vi "SMS Analysis Interface.vi"(7 "Calling VI Ref":refnum<vi>) -> ()   [LabVIEW 2016]
uses:
  <vilib>/Utility/miscctls.llb/LVPointTypeDef.ctl
  Orca Flash Data Spooler/Orca Data Spooler Type Defs/Orca Data Spooler Transfer Data.ctl
  SMS Analysis Interface Type Defs/SMS Analysis Interface Connection Info.ctl
panel:
  in  "Clear Queue":bool
  out "Connection Error":bool
  out "Remote Running":bool
  out "Remote Ready":bool
  in  "Queue List":i32(listbox)
  in  "Pause Queue":bool
  in  "Quit Remote":bool
  in  "Add Dataset":bool
  in  "Quit":bool
  out "Start Up Error":errorcluster
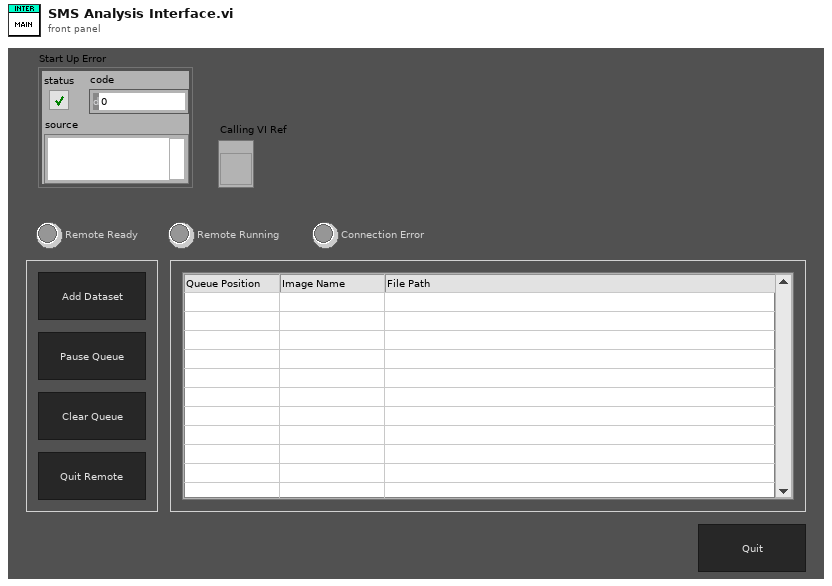
[diagram p1: front panel]
types:
  T1 = typedef "SMS Analysis Interface Connection Info.ctl" = cluster{"Remote IP":string, "Port":u16}
  T2 = typedef "Orca Data Spooler Transfer Data.ctl" = cluster{"transLogPath":string, "imageName":string, "noFrames":u32, "noCycles":u16, "quitFlag":bool}
  T3 = enum16{"Always On", "Always Off", "Off While Running"}
  T4 = typedef "LVPointTypeDef.ctl" = cluster{"Horizontal":i16, "Vertical":i16}
  T5 = typedef "LVRectTypeDef.ctl" = cluster{"Left":i16, "Top":i16, "Right":i16, "Bottom":i16}
  T6 = typedef "LVBoundsTypeDef.ctl" = cluster{"Width":u32, "Height":u32}
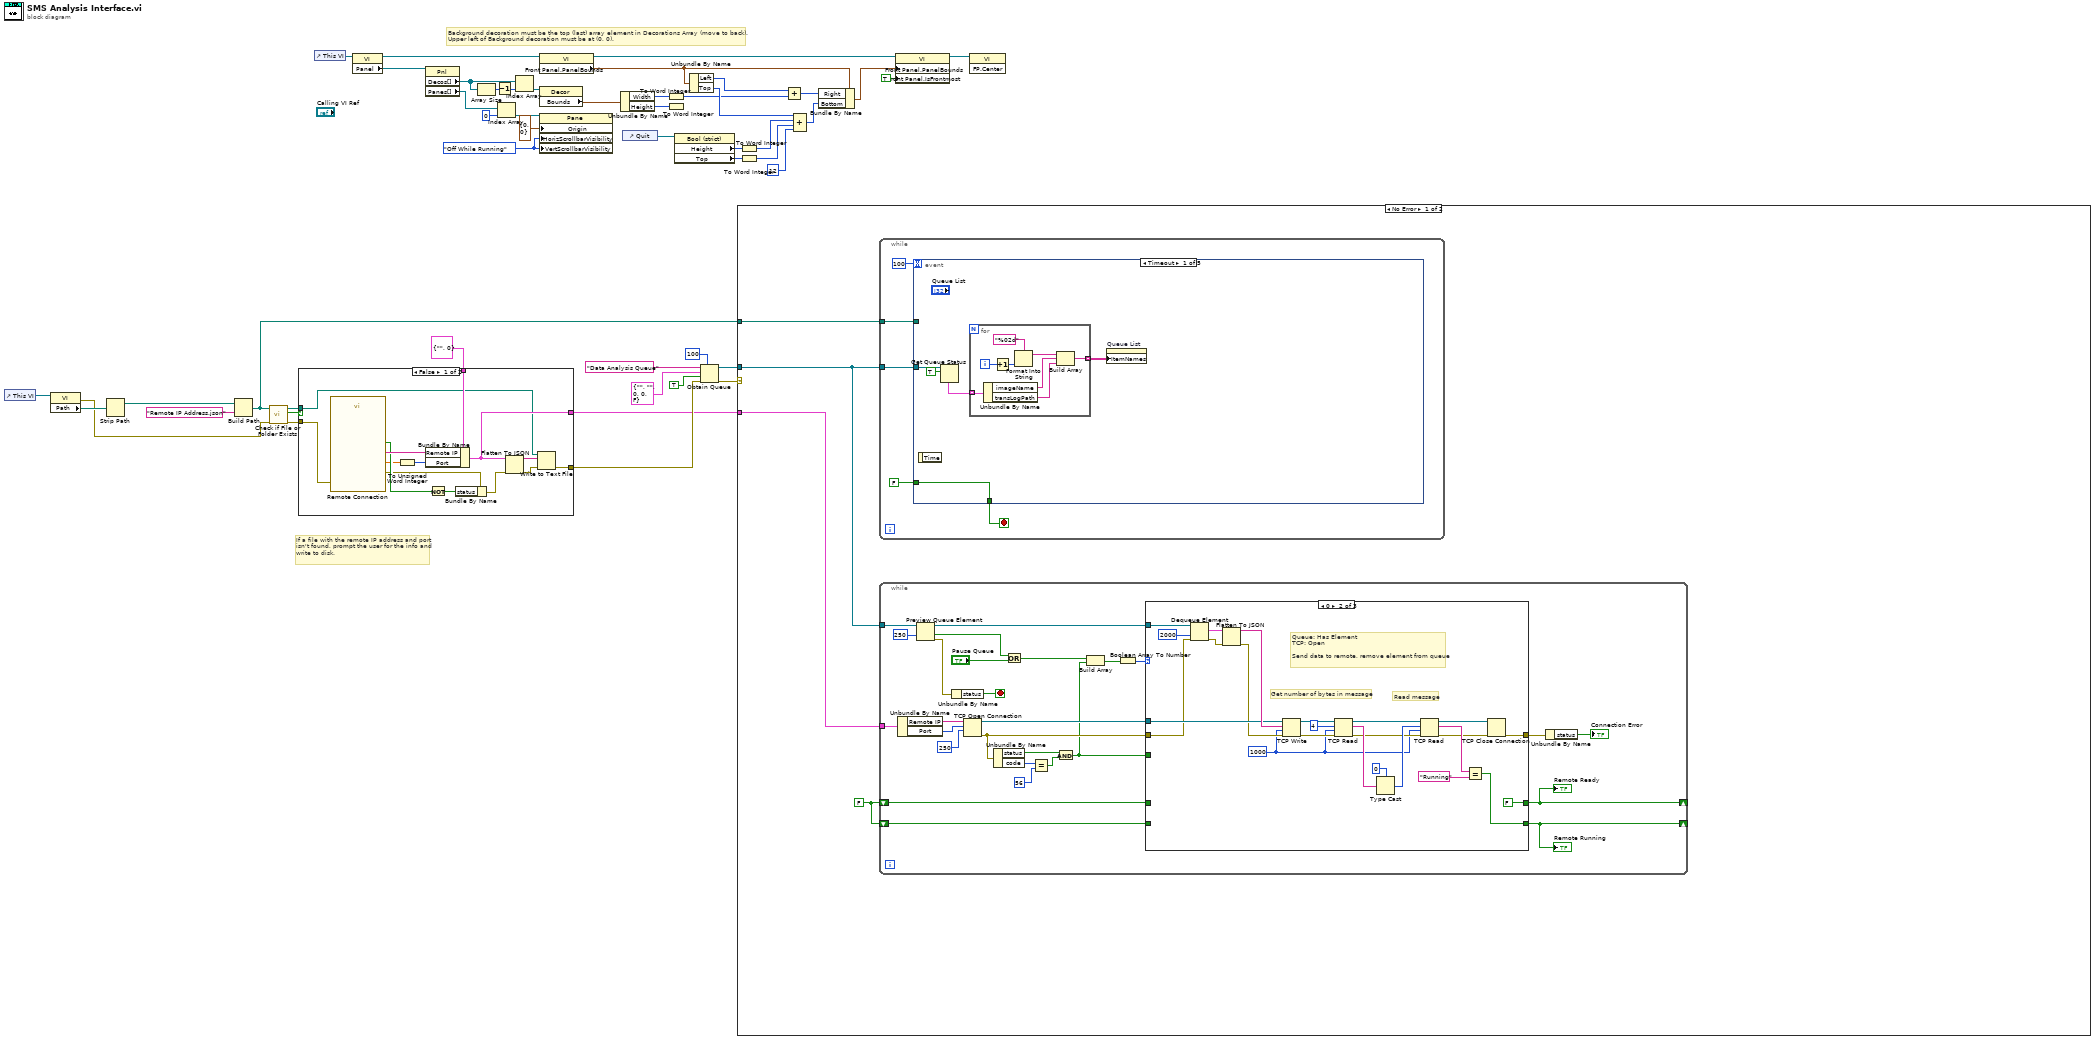
[diagram p0: block diagram]
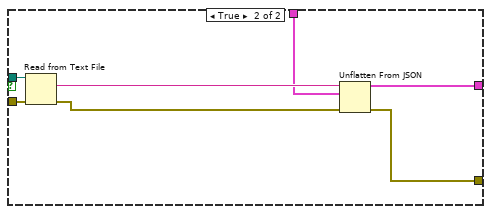
[diagram p2: hidden frame]
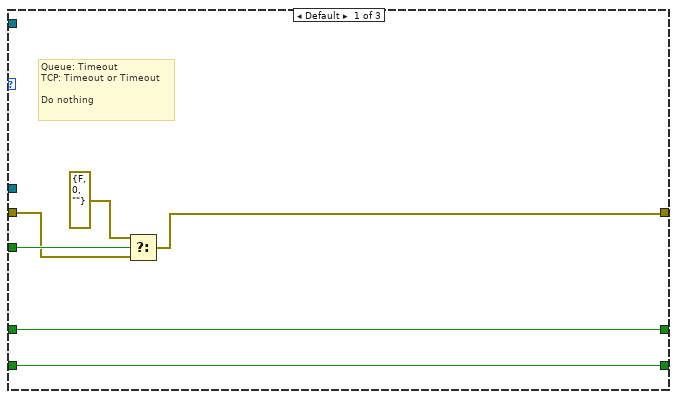
[diagram p3: hidden frame]
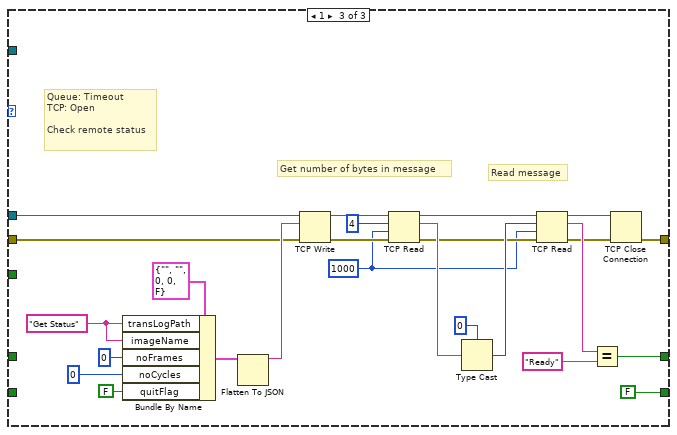
[diagram p4: hidden frame]
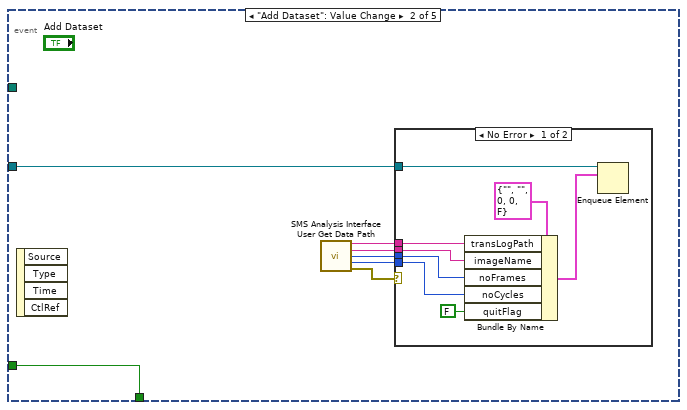
[diagram p5: hidden frame]
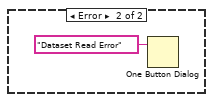
[diagram p6: hidden frame]
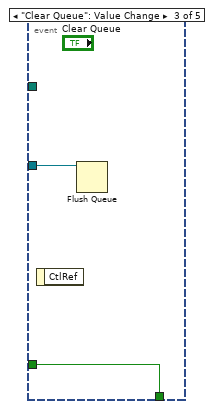
[diagram p7: hidden frame]
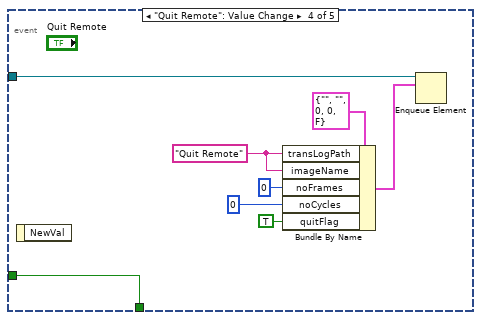
[diagram p8: hidden frame]
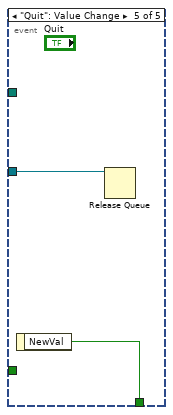
[diagram p9: hidden frame]
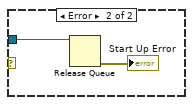
[diagram p10: hidden frame]
diagram:
  w26 = T3."Off While Running" ("Vertical Scrollbar Visibility")
  # "If a file with the remote IP address and port isn't found, prompt the user for the info and write to disk."
  # "Background decoration must be the top (last) array element in Decorations Array (move to back).\nUpper left of Background decoration must be at (0, 0)."
  n1 = control-ref of="This VI"() -> (w49:refnum<vi>)
  n2 = property class="VI"(reference=w49) -> (error out=w5:errorcluster, "Path"=w48:path)  [unwired: 1 in, 1 out]
  n3 = Strip Path(path=w48) -> (stripped path=w46:path)  [unwired: 1 out]
  n4 = Build Path(base path=w46, name or relative path="Remote IP Address.json" ("name (unnamed)")) -> (appended path=w14:path)
  n5 = call <vilib>:"Check if File or Folder Exists.vi"("error in (no error)"=w5, "path"=w14) -> ("error out"=w6:errorcluster, "file or folder exists?"=w44:bool, "dup path"=w45:path)  [unwired: 7 in]
  n6 = case shown="False" w44 {
    tunnel: w45 -> [w56 w68]
    tunnel: [w62 w67] -> w1
    tunnel: T1 {"Remote IP"="", "Port"=0} ("Connection Data") -> [w63 w66]
    tunnel: [w57 w64] -> w4
    tunnel: w6 -> [w54 w65]
    frame False {
      n7 = call "Remote Connection"("error in (no error)"=w54) -> ("Port"=w51:dbl, "IP Address"=w55:string, "OK"=w53:bool, "error out"=w52:errorcluster)  [unwired: 15 in]
      n8 = To Unsigned Word Integer(number=w51) -> (unsigned 16bit integer=w50:u16)
      n9 = Bundle By Name(cluster=w63, "Remote IP"=w55, "Port"=w50) -> (w62:T1)
      n10 = Not(x=w53) -> (.not. x?=w59:bool)
      n11 = Bundle By Name(cluster=w52, "status"=w59) -> (w58:errorcluster)
      n12 = Flatten To JSON(anything=w62, error in (no error)=w58) -> (JSON string=w61:string, 11:w60:errorcluster)  [unwired: 1 in]
      n13 = Write to Text File(file (use dialog)=w56, text=w61, error in=w60) -> (error out=w57:errorcluster)  [unwired: 1 in, 2 out]
    }
    frame True {
      n14 = Read from Text File(file (use dialog)=w68, error in=w65) -> (text=w70:string, error out=w69:errorcluster)  [unwired: 2 in, 2 out]
      n15 = Unflatten From JSON(JSON string=w70, type and defaults=w66, error in (no error)=w69) -> (value=w67:T1, error out=w64:errorcluster)  [unwired: 4 in]
    }
  }
  n16 = control-ref of="This VI"() -> (w18:refnum<vi>)
  n17 = property class="VI"(reference=w18) -> (reference out=w27:refnum<vi>, "Panel"=w19:refnum<vi>)  [unwired: 1 in, 1 out]
  n18 = property class="Pnl"(reference=w19) -> ("Decos[]"=w17:refnum<vi>[], "Panes[]"=w23:refnum<vi>[])  [unwired: 1 in, 2 out]
  n19 = Array Size(array=w17) -> (size(s)=w15:i32)
  n20 = Decrement(x=w15) -> (x-1=w16:i32)
  n21 = Index Array(array=w23, index=0) -> (element=w22:refnum<vi>)
  n22 = Index Array(array=w17, index=w16) -> (element=w25:refnum<vi>)
  n23 = property class="VI"(reference=w27) -> (reference out=w29:refnum<vi>, "Front Panel.PanelBounds"=w30:T5)  [unwired: 1 in, 1 out]
  n24 = property class="Decor"(reference=w25) -> ("Bounds"=w28:T6)  [unwired: 1 in, 2 out]
  n25 = property class="Pane"(reference=w22, "Origin"=T4 {"Horizontal"=0, "Vertical"=0}, "HorizScrollbarVisibility"=w26, "VertScrollbarVisibility"=w26) -> ()  [unwired: 1 in, 2 out]
  n26 = Unbundle By Name(w28) -> ("Width"=w33:u32, "Height"=w36:u32)
  n27 = control-ref of="Quit"() -> (w20:refnum<vi>)
  n28 = To Word Integer(number=w33) -> (16bit integer=w35:i16)
  n29 = To Word Integer(number=w36) -> ()  [unwired: 1 out]
  n30 = property class="Bool (strict)"(reference=w20) -> ("Height"=w38:u32, "Top"=w39:i32)  [unwired: 1 in, 2 out]
  n31 = Unbundle By Name(w30) -> ("Left"=w32:i16, "Top"=w43:i16)
  n32 = Obtain Queue(max queue size (-1, unlimited)=100, name (unnamed)="Data Analysis Queue", element data type=T2 {"transLogPath"="", "imageName"="", "noFrames"=0, "noCycles"=0, "quitFlag"=FALSE} ("Spooler Connection Data"), create if not found? (T)=TRUE, error in (no error)=w4) -> (queue out=w9:refnum<queue>, error out=w8:errorcluster)  [unwired: 1 out]
  n33 = case shown="No Error" w8 {
    tunnel: w14 -> [w74 _]
    tunnel: w9 -> [w73 w204]
    tunnel: w1 -> [w72 _]
    frame No Error {
      w71 = FALSE
      n34 = while {
        tunnel: w74 -> [w158]
        tunnel: w73 -> [w157]
        stop <- w160 stop-if-true
        n35 = event shown="[0] Timeout" {
          selector: _ -> [_ _ _ _ _]
          dyn-events: _ -> [_ _ _ _ _]
          timeout: 100 -> [_ _ _ _ _]
          tunnel: FALSE -> [w166 w181 w192 w200 _]
          tunnel: [w166 w181 w192 w200 w202] -> w160
          tunnel: w158 -> [_ _ _ _ _]
          tunnel: w157 -> [w165 w180 w191 w193 w201]
          event Timeout {
            n36 = event-data() -> ()  [unwired: 1 in, 1 out]
            n37 = Get Queue Status(queue=w165, return elements? (F)=TRUE) -> (elements=w164:T2[])  [unwired: 1 in, 7 out]
            n38 = for {
              tunnel: w164 -> [w174] mode=indexing
              tunnel: [w168] -> w162 mode=indexing
              i -> [w172]
              n39 = Unbundle By Name(w174) -> ("imageName"=w170:string, "transLogPath"=w169:string)
              n40 = Increment(x=w172) -> (x+1=w167:i32)
              n41 = Format Into String(format string="%02d", w167) -> (resulting string=w171:string)  [unwired: 2 in, 1 out]
              n42 = Build Array(w171, w170, w169) -> (w168:string[])
            }
            n43 = property on="Queue List" class="MCListbox (strict)"("ItemNames"=w162) -> ()  [unwired: 2 in, 2 out]
          }
          event "Add Dataset": Value Change {
            n44 = event-data() -> ()  [unwired: 1 in, 4 out]
            n45 = call "SMS Analysis Interface User Get Data Path.vi"() -> ("Transfer Log Path"=w179:string, "Image Name"=w178:string, "Frames"=w177:u32, "Cycles"=w176:u16, "Error"=w175:errorcluster)  [unwired: 11 in]
            n46 = case shown="No Error" w175 {
              tunnel: w180 -> [w187 _]
              tunnel: w179 -> [w185 _]
              tunnel: w178 -> [w184 _]
              tunnel: w177 -> [w183 _]
              tunnel: w176 -> [w182 _]
              frame No Error {
                n47 = Bundle By Name(cluster=T2 {"transLogPath"="", "imageName"="", "noFrames"=0, "noCycles"=0, "quitFlag"=FALSE} ("Spooler Connection Data"), "transLogPath"=w185, "imageName"=w184, "noFrames"=w183, "noCycles"=w182, "quitFlag"=FALSE) -> (w186:T2)
                n48 = Enqueue Element(queue=w187, element=w186) -> ()  [unwired: 2 in, 3 out]
              }
              frame Error {
                n49 = One Button Dialog(message="Dataset Read Error") -> ()  [unwired: 1 in, 1 out]
              }
            }
          }
          event "Clear Queue": Value Change {
            n50 = event-data() -> ()  [unwired: 1 in, 1 out]
            n51 = Flush Queue(queue=w191) -> ()  [unwired: 1 in, 3 out]
          }
          event "Quit Remote": Value Change {
            w194 = "Quit Remote" ("transLogPath")
            n52 = event-data() -> ()  [unwired: 1 in, 1 out]
            n53 = Bundle By Name(cluster=T2 {"transLogPath"="", "imageName"="", "noFrames"=0, "noCycles"=0, "quitFlag"=FALSE} ("Spooler Connection Data"), "transLogPath"=w194, "imageName"=w194, "noFrames"=u32 0, "noCycles"=u16 0, "quitFlag"=TRUE) -> (w197:T2)
            n54 = Enqueue Element(queue=w193, element=w197) -> ()  [unwired: 2 in, 3 out]
          }
          event "Quit": Value Change {
            n55 = event-data() -> ("NewVal"=w202:bool)  [unwired: 1 in]
            n56 = Release Queue(queue=w201) -> ()  [unwired: 2 in, 3 out]
          }
        }
      }
      n57 = while {
        tunnel: w73 -> [w101]
        tunnel: w72 -> [w97]
        shift-right: [w77] -> _
        shift-left: w71 -> [w80]
        shift-right: [w78] -> _
        shift-left: w71 -> [w79]
        stop <- w98 stop-if-true
        n58 = Unbundle By Name(w97) -> ("Remote IP"=w96:string, "Port"=w95:u16)
        n59 = Preview Queue Element(queue=w101, timeout in ms (-1)=250) -> (queue out=w84:refnum<queue>, timed out?=w94:bool, error out=w99:errorcluster)  [unwired: 1 in, 1 out]
        n60 = Unbundle By Name(w99) -> ("status"=w98:bool)
        n61 = TCP Open Connection(address=w96, remote port or service name=w95, timeout ms (60000)=250) -> (connection ID=w86:refnum<k5>, error out=w85:errorcluster)  [unwired: 2 in]
        n62 = Unbundle By Name(w85) -> ("status"=w88:bool, "code"=w91:i32)
        n63 = Or(x=w94, y="Pause Queue") -> (x .or. y?=w83:bool)
        n64 = Equal?(x=w91, y=56) -> (x = y?=w87:bool)
        n65 = And(x=w88, y=w87) -> (x .and. y?=w75:bool)
        n66 = Build Array(w83, w75) -> (w82:bool[])
        n67 = Boolean Array To Number(Boolean array=w82) -> (number=w81:u32)
        n68 = case shown="0" w81 {
          tunnel: w86 -> [_ w119 w150]
          tunnel: w85 -> [w104 w116 w140]
          tunnel: [w102 w108 w132] -> w76
          tunnel: w84 -> [_ w131 _]
          tunnel: w80 -> [w107 _ _]
          tunnel: w79 -> [w106 _ _]
          tunnel: [w107 FALSE w136] -> w77
          tunnel: [w106 w112 FALSE] -> w78
          tunnel: w75 -> [w105 _ _]
          frame Default {
            # "Queue: Timeout\nTCP: Timeout or Timeout\n\nDo nothing"
            n69 = Select(t=errorcluster {"status"=FALSE, "code"=0, "source"=""} ("error out"), s=w105, f=w104) -> (s? t:f=w102:errorcluster)
          }
          frame 0 {
            w113 = 1000 ("timeout ms (25000)")
            # "Read message"
            # "Get number of bytes in message"
            # "Queue: Has Element\nTCP: Open\n\nSend data to remote, remove element from queue"
            n70 = Dequeue Element(queue=w131, timeout in ms (-1)=2000, error in (no error)=w116) -> (element=w118:T2, error out=w117:errorcluster)  [unwired: 2 out]
            n71 = Flatten To JSON(anything=w118, error in (no error)=w117) -> (JSON string=w130:string, 11:w114:errorcluster)  [unwired: 1 in]
            n72 = TCP Write(connection ID=w119, data in=w130, error in (no error)=w114, 9:w113) -> (connection ID out=w129:refnum<k5>, error out=w123:errorcluster)  [unwired: 1 out]
            n73 = TCP Read(connection ID=w129, bytes to read=4, error in (no error)=w123, 9:w113) -> (connection ID out=w125:refnum<k5>, data out=w126:string, error out=w122:errorcluster)  [unwired: 1 in]
            n74 = Type Cast(type=0 ("timeout ms (25000)"), x=w126) -> (*(type *) &x=w124:i32)
            n75 = TCP Read(connection ID=w125, bytes to read=w124, error in (no error)=w122, 9:w113) -> (connection ID out=w110:refnum<k5>, data out=w121:string, error out=w109:errorcluster)  [unwired: 1 in]
            n76 = Equal?(x=w121, y="Running") -> (x = y?=w112:bool)
            n77 = TCP Close Connection(connection ID=w110, error in (no error)=w109) -> (error out=w108:errorcluster)  [unwired: 1 in, 1 out]
          }
          frame 1 {
            w137 = 1000 ("timeout ms (25000)")
            w155 = "Get Status" ("transLogPath")
            # "Queue: Timeout\nTCP: Open\n\nCheck remote status"
            # "Read message"
            # "Get number of bytes in message"
            n78 = Bundle By Name(cluster=T2 {"transLogPath"="", "imageName"="", "noFrames"=0, "noCycles"=0, "quitFlag"=FALSE} ("Spooler Connection Data"), "transLogPath"=w155, "imageName"=w155, "noFrames"=u32 0, "noCycles"=u16 0, "quitFlag"=FALSE) -> (w156:T2)
            n79 = Flatten To JSON(anything=w156) -> (JSON string=w149:string)  [unwired: 2 in, 1 out]
            n80 = TCP Write(connection ID=w150, data in=w149, error in (no error)=w140) -> (connection ID out=w148:refnum<k5>, error out=w142:errorcluster)  [unwired: 1 in, 1 out]
            n81 = TCP Read(connection ID=w148, bytes to read=4, error in (no error)=w142, 9:w137) -> (connection ID out=w144:refnum<k5>, data out=w145:string, error out=w141:errorcluster)  [unwired: 1 in]
            n82 = Type Cast(type=0 ("timeout ms (25000)"), x=w145) -> (*(type *) &x=w143:i32)
            n83 = TCP Read(connection ID=w144, bytes to read=w143, error in (no error)=w141, 9:w137) -> (connection ID out=w134:refnum<k5>, data out=w139:string, error out=w133:errorcluster)  [unwired: 1 in]
            n84 = Equal?(x=w139, y="Ready") -> (x = y?=w136:bool)
            n85 = TCP Close Connection(connection ID=w134, error in (no error)=w133) -> (error out=w132:errorcluster)  [unwired: 1 in, 1 out]
          }
        }
        "Remote Ready" <- w77
        "Remote Running" <- w78
        n86 = Unbundle By Name(w76) -> ("status"=→"Connection Error":bool)
      }
    }
    frame Error {
      n87 = Release Queue(queue=w204) -> (error out=→"Start Up Error":errorcluster)  [unwired: 2 in, 2 out]
    }
  }
  n88 = To Word Integer(number=w38) -> (16bit integer=w41:i16)
  n89 = To Word Integer(number=w39) -> (16bit integer=w42:i16)
  n90 = Add(x=w32, y=w35) -> (x+y=w34:i16)
  n91 = Compound Arithmetic op=ADD(w43, w41, w42, i16 12 ("y")) -> (w37:i16)
  n92 = Bundle By Name(cluster=w30, "Right"=w34, "Bottom"=w37) -> (w31:T5)
  n93 = property class="VI"(reference=w29, "Front Panel.PanelBounds"=w31, "Front Panel.IsFrontmost"=TRUE ("Front Panel Window:Is Frontmost")) -> (reference out=w3:refnum<vi>)  [unwired: 1 in, 1 out]
  n94 = invoke class="VI" method="FP.Center"(reference=w3) -> ()  [unwired: 2 in, 3 out]
